vi "Quadcopter.vi"(11 "Z":sgl) -> ()   [LabVIEW 2013]
uses:
  <vilib>/Utility/miscctls.llb/LV3DPointTypeDef.ctl
  <vilib>/picture/3D Picture Control/Object/Create Object (name).vi
  <vilib>/picture/3D Picture Control/Object/Add Object (no reference).vi
  <vilib>/picture/3D Picture Control/Object/Add Object (reference).vi
  <vilib>/picture/3D Picture Control/NI_3D Picture Control.lvlib
panel:
  out "floor(x/y) 2":dbl
  in  "Propellers 2":path=path "D:/CELLUM/QuadDemo/3D Model/PropellerGreen.wrl"
  in  "Propellers":path=path "D:/CELLUM/QuadDemo/3D Model/Propeller.wrl"
  in  "Y":dbl(slide) scale=-10.0..10.0
  in  "X":dbl(slide) scale=-10.0..10.0
  in  "Roll":dbl(knob) scale=0.0..360.0
  in  "stop":bool
  in  "Body":path=path "D:/CELLUM/QuadDemo/3D Model/Body.wrl"
  out "error out":errorcluster
  out "3D Picture":refnum<vi>(3d-picture)
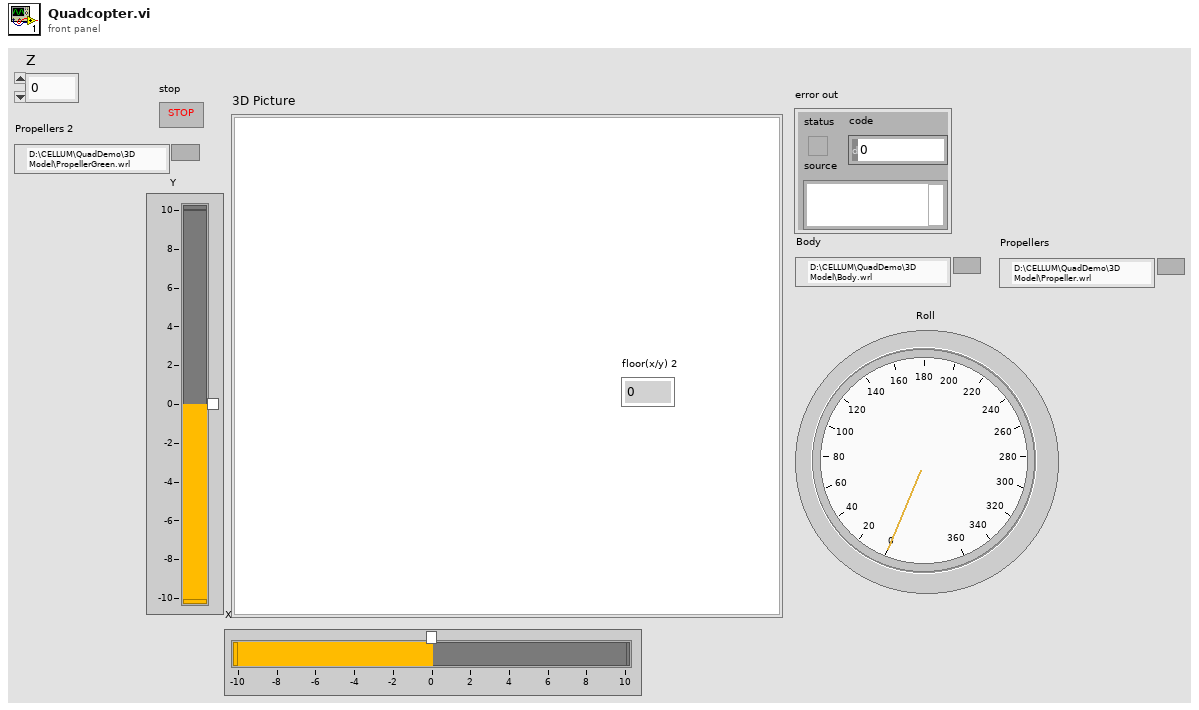
[diagram p1: front panel]
types:
  T1 = typedef "LV3DPointTypeDef.ctl" = cluster{"X":sgl, "Y":sgl, "Z":sgl}
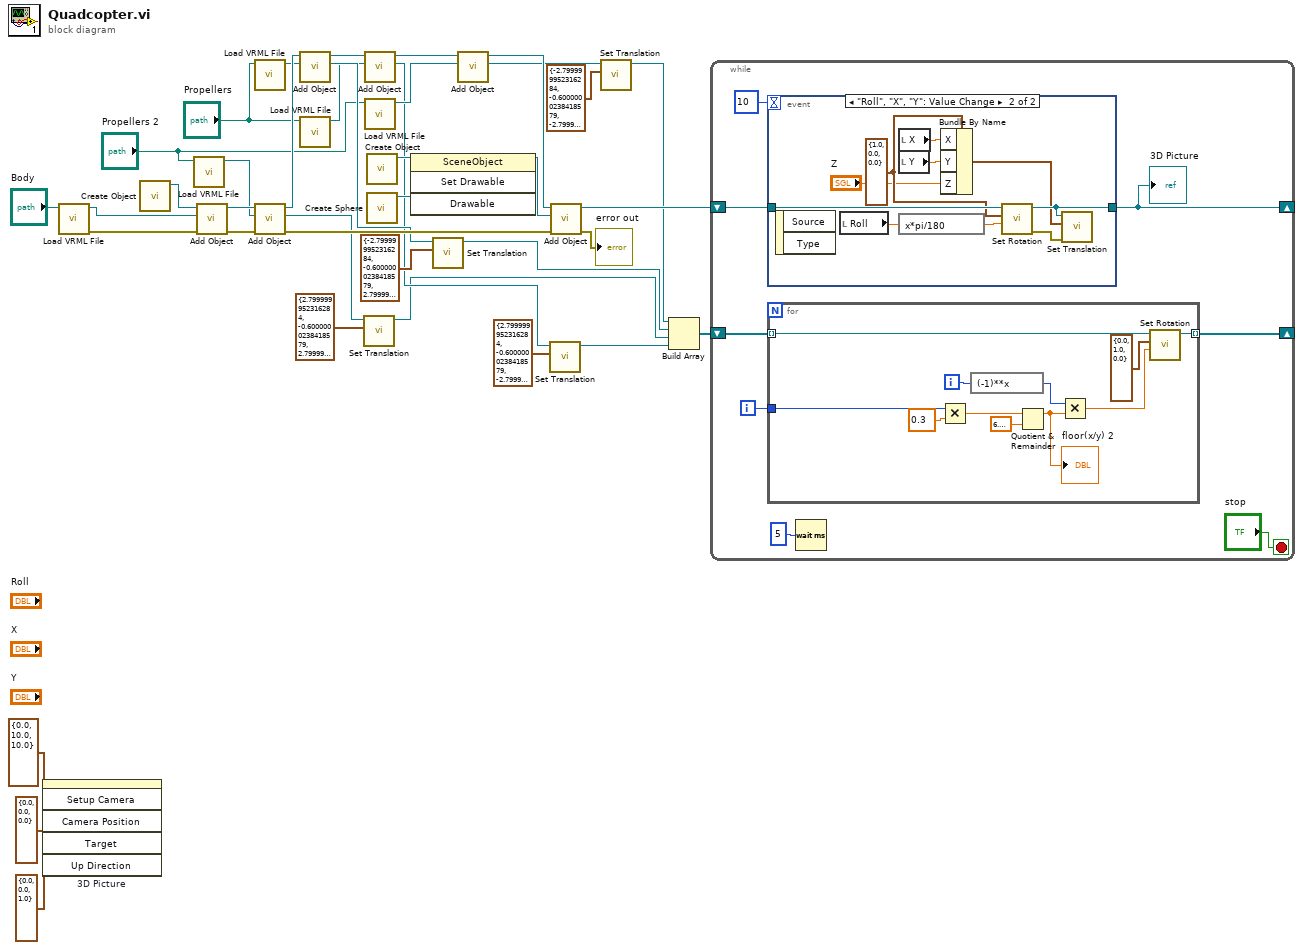
[diagram p0: block diagram]
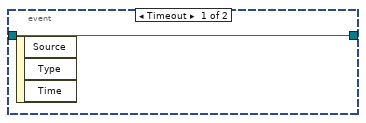
[diagram p2: hidden frame]
diagram:
  n1 = invoke on="3D Picture" class="SceneGraphDisp (strict)" method="Setup Camera"("Camera Position"=T1 {"X"=0.0, "Y"=10.0, "Z"=10.0}, "Target"=T1 {"X"=0.0, "Y"=0.0, "Z"=0.0}, "Up Direction"=T1 {"X"=0.0, "Y"=0.0, "Z"=1.0}) -> ()  [unwired: 3 in, 6 out]
  n2 = call <vilib>:"Load VRML File.vi"("Path"="Body") -> ("error out"=w36:errorcluster, "Scene:Read Scene File"=w37:refnum<vi>)  [unwired: 9 in]
  n3 = call-poly <vilib>:"Create Object.vi"() -> ("Scene:New Object"=w38:refnum<vi>)  [unwired: 10 in, 1 out]
  n4 = call <vilib>:"Load VRML File.vi"("Path"="Propellers 2") -> ("Scene:Read Scene File"=w20:refnum<vi>)  [unwired: 9 in, 1 out]
  n5 = call-poly <vilib>:"Add Object.vi"("error in (no error)"=w36, "New Object In"=w37, "Scene Object In"=w38) -> ("error out"=w25:errorcluster, "Scene Object Out"=w26:refnum<vi>)  [unwired: 7 in]
  n6 = call <vilib>:"Load VRML File.vi"("Path"="Propellers") -> ("Scene:Read Scene File"=w19:refnum<vi>)  [unwired: 9 in, 1 out]
  n7 = call-poly <vilib>:"Add Object.vi"("error in (no error)"=w25, "New Object In"=w20, "Scene Object In"=w26) -> ("error out"=w24:errorcluster, "New Object Out"=w23:refnum<vi>, "Scene Object Out"=w21:refnum<vi>)  [unwired: 6 in]
  n8 = call-poly <vilib>:"Add Object.vi"("New Object In"=w19, "Scene Object In"=w21) -> ("New Object Out"=w17:refnum<vi>, "Scene Object Out"=w12:refnum<vi>)  [unwired: 7 in, 1 out]
  n9 = call <vilib>:"Load VRML File.vi"("Path"="Propellers") -> ("Scene:Read Scene File"=w11:refnum<vi>)  [unwired: 9 in, 1 out]
  n10 = call <vilib>:"Set Translation.vi"("Translation"=cluster{"X":sgl, "Y":sgl, "Z":sgl} {"X"=2.8, "Y"=-0.6, "Z"=2.8}, "Scene Object"=w23) -> ("Translated Object"=w1:refnum<vi>)  [unwired: 8 in, 1 out]
  n11 = call-poly <vilib>:"Add Object.vi"("New Object In"=w11, "Scene Object In"=w12) -> ("New Object Out"=w9:refnum<vi>, "Scene Object Out"=w10:refnum<vi>)  [unwired: 7 in, 1 out]
  n12 = call <vilib>:"Load VRML File.vi"("Path"="Propellers 2") -> ("Scene:Read Scene File"=w15:refnum<vi>)  [unwired: 9 in, 1 out]
  n13 = call-poly <vilib>:"Create Object.vi"() -> ("Scene:New Object"=w28:refnum<vi>)  [unwired: 10 in, 1 out]
  n14 = call <vilib>:"Create Sphere.vi"() -> ("New Sphere Refnum"=w29:refnum<vi>)  [unwired: 10 in, 1 out]
  n15 = invoke class="SceneObject" method="Set Drawable"(reference=w28, "Drawable"=w29) -> (reference out=w27:refnum<vi>)  [unwired: 2 in, 3 out]
  n16 = call <vilib>:"Set Translation.vi"("Translation"=cluster{"X":sgl, "Y":sgl, "Z":sgl} {"X"=-2.8, "Y"=-0.6, "Z"=2.8}, "Scene Object"=w17) -> ("Translated Object"=w2:refnum<vi>)  [unwired: 8 in, 1 out]
  n17 = call-poly <vilib>:"Add Object.vi"("New Object In"=w15, "Scene Object In"=w10) -> ("New Object Out"=w13:refnum<vi>, "Scene Object Out"=w14:refnum<vi>)  [unwired: 7 in, 1 out]
  n18 = call <vilib>:"Set Translation.vi"("Translation"=cluster{"X":sgl, "Y":sgl, "Z":sgl} {"X"=2.8, "Y"=-0.6, "Z"=-2.8}, "Scene Object"=w9) -> ("Translated Object"=w3:refnum<vi>)  [unwired: 8 in, 1 out]
  n19 = call-poly <vilib>:"Add Object.vi"("error in (no error)"=w24, "New Object In"=w27, "Scene Object In"=w14) -> ("error out"=→"error out":errorcluster, "Scene Object Out"=w31:refnum<vi>)  [unwired: 7 in]
  n20 = call <vilib>:"Set Translation.vi"("Translation"=cluster{"X":sgl, "Y":sgl, "Z":sgl} {"X"=-2.8, "Y"=-0.6, "Z"=-2.8}, "Scene Object"=w13) -> ("Translated Object"=w5:refnum<vi>)  [unwired: 8 in, 1 out]
  n21 = Build Array(w5, w2, w1, w3) -> (w4:refnum<vi>[])
  n22 = while {
    shift-right: [w43] -> _
    shift-left: w31 -> [w44]
    shift-right: [w40] -> _
    shift-left: w4 -> [w41]
    i -> [w39]
    stop <- "stop" stop-if-true
    n23 = event shown="[1] \"Roll\", \"X\", \"Y\": Value Change" {
      selector: _ -> [_ _]
      dyn-events: _ -> [_ _]
      timeout: 10 -> [_ _]
      tunnel: w44 -> [w58 w68]
      tunnel: [w58 w65] -> w43
      event Timeout {
        n24 = event-data() -> ()  [unwired: 1 in, 3 out]
      }
      event "Roll", "X", "Y": Value Change {
        w63 = cluster{"X":sgl, "Y":sgl, "Z":sgl} {"X"=1.0, "Y"=0.0, "Z"=0.0} ("Axis")
        n25 = event-data() -> ()  [unwired: 1 in, 2 out]
        n26 = local read "Roll"() -> (w64:dbl)
        n27 = local read "X"() -> (w61:dbl)
        n28 = local read "Y"() -> (w60:dbl)
        n29 = expression code="x*pi/180"(w64) -> (w67:dbl)
        n30 = Bundle By Name(cluster=w63, "X"=w61, "Y"=w60, "Z"="Z") -> (w62:cluster{"X":sgl, "Y":sgl, "Z":sgl})
        n31 = call <vilib>:"Set Rotation.vi"("Angle"=w67, "Axis"=w63, "Scene Object"=w68) -> ("error out"=w66:errorcluster, "Rotated Scene Object"=w65:refnum<vi>)  [unwired: 7 in]
        n32 = call <vilib>:"Set Translation.vi"("error in (no error)"=w66, "Translation"=w62, "Scene Object"=w65) -> ()  [unwired: 7 in, 2 out]
      }
    }
    "3D Picture" <- w43
    n33 = for {
      tunnel: w41 -> [w54] mode=indexing
      tunnel: [w53] -> w40 mode=indexing
      tunnel: w39 -> [w51]
      i -> [w48]
      n34 = Multiply(x=w51, y=0.3) -> (x*y=w49:dbl)
      n35 = expression code="(-1)**x"(w48) -> (w47:i32)
      n36 = Quotient & Remainder(x=w49, y=6.283185307179586) -> (x-y*floor(x/y)=w57:dbl)  [unwired: 1 out]
      "floor(x/y) 2" <- w57
      n37 = Multiply(x=w47, y=w57) -> (x*y=w50:dbl)
      n38 = call <vilib>:"Set Rotation.vi"("Angle"=w50, "Axis"=cluster{"X":sgl, "Y":sgl, "Z":sgl} {"X"=0.0, "Y"=1.0, "Z"=0.0}, "Scene Object"=w54) -> ("Rotated Scene Object"=w53:refnum<vi>)  [unwired: 7 in, 1 out]
    }
    n39 = Wait (ms)(milliseconds to wait=u32 5) -> ()  [unwired: 1 out]
  }
